vi "Parse XML Heap.vi"(8 "Error in":errorcluster caption="Error in (no error)", 11 "XML":string) -> (0 "Error out":errorcluster, 3 "Root Element":refnum<class "Attribute.lvclass">)   [LabVIEW 2018, in "VILab.lvlib"]
uses:
  VILab.lvlib
  Attribute.lvclass
  <vilib>/xml/Load XML String.vi
  <vilib>/xml/Close Reference(Node).vi
  <vilib>/xml/NI_XML.lvlib
  <resource>/objmgr/DOMUserDefRef.rc
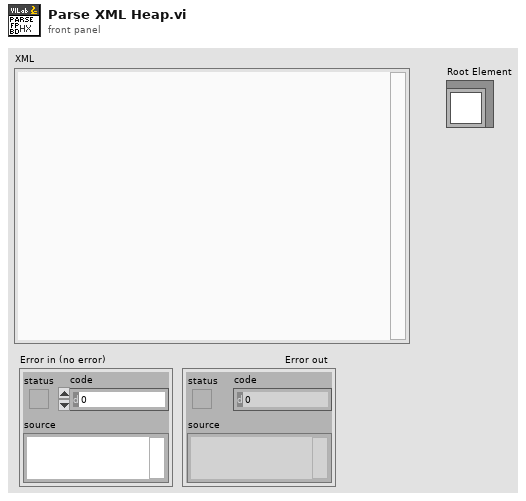
[diagram p1: front panel]
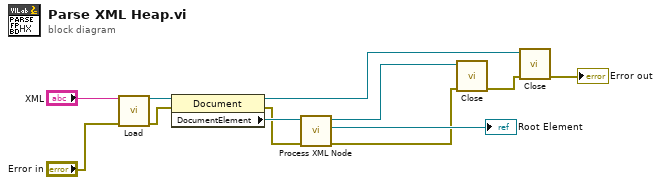
[diagram p0: block diagram]
diagram:
  n1 = call-poly <vilib>:"Load.vi"("XML string"="XML", "error in (no error)"="Error in") -> ("DOM document out"=w10:refnum<k20>, "error out"=w8:errorcluster)  [unwired: 11 in, 1 out]
  n2 = property class="Document"(reference=w10, error in=w8) -> (reference out=w5:refnum<k20>, error out=w7:errorcluster, "DocumentElement"=w9:refnum<k20>)
  n3 = call "Process XML Node.vi"("Error in"=w7, "XML Element"=w9) -> ("Error out"=w1:errorcluster, "Attribute"=→"Root Element":refnum<class "Attribute.lvclass">, "XML Element Out"=w6:refnum<k20>)  [unwired: 7 in]
  n4 = call-poly <vilib>:"Close.vi"("error in (no error)"=w1, "node"=w6) -> ("error out"=w3:errorcluster)  [unwired: 7 in]
  n5 = call-poly <vilib>:"Close.vi"("error in (no error)"=w3, "node"=w5) -> ("error out"=→"Error out":errorcluster)  [unwired: 7 in]
